vi "mag-field_wait_field.vi"(10 "instr params":T1={"DACs info"={"FPGA VI Reference"=refnum, "Delay"=0, "Last known values"=[], "sent values"=[], "Secured gate"=[], "lock-in config"={"channel (cl)"={"panel LI"=0, "channel LI"=0}, "frequency (Hz)"=0.0, "amplitude (V)"=0.0}, "DAC_Connection"={"DAC"=[], "DAC_Number"=0.0}}, "AWG 8257"={"RF parms"={"Freq(GHz)"={"from"=0.0, "to"=0.0, "String"="", "type"=enum."static"}, "Ampl(dBm)"={"from"=0.0, "to"=0.0, "String"="", "type"=enum."static"}}, "RF on?"=FALSE, "RF info"={"RF freq"=0.0, "RF pow"=0.0, "On?"=FALSE}, "GPIB adr"="", "Activate?"=FALSE, "use System decimal point"=FALSE, "way_of_connection"=0, "VISA_address"=""}, "mag fiel params"={"mag field"={"from"=0.0, "to"=0.0, "type"=enum."static"}, "use perm mode"=FALSE, "field info out"={"B field (consigne)"=0.0, "B field"=0.0, "B-field driver (vi reference)"=refnum, "consigne ctrl (driver)"=refnum, "field has arrived (ctrl, driver)"=refnum, "field  (ctrl, driver)"=refnum, "Coil supply"=refnum, "GPIB adress"=refnum}, "GPIB adr"="", "driver running?"=FALSE, "ON?"=FALSE, "Coil_Information"={"Max Field 10V Input"=0.0, "Waiting time for 0.5mT step"=0.0, "Dac_Output_Channel"=""}}, "K2000 - 01"={"Range (V) 2"="", "Digits 2"="", "NPLC"="", "NPLC fast"="", "GPIB Address"="", "average"=0, "GPIB - PAD"=0, "Use K2000?"=FALSE}, "K2000 - 02"={"Range (V) 2"="", "Digits 2"="", "NPLC"="", "NPLC fast"="", "GPIB Address"="", "average"=0, "GPIB - PAD"=0, "Use K2000?"=FALSE}, "LeCroy6050A"={"LeCroy6050A"={"VISA resource name"="", "Sources"={"Source 1"={"S1_actived"=FALSE, "Source1"=0}, "Source 2"={"S1_actived"=FALSE, "Source1"=0}, "Source 3"={"S1_actived"=FALSE, "Source1"=0}, "Source 4"={"S1_actived"=FALSE, "Source1"=0}}, "Use LeCroy"=FALSE, "time/div"=0.0, "sampling rate"=0.0}, "Activated channels"=[]}, "fast sequence"={"fast channels"={"fast channel 0"={"panel"=0, "chanel"=0, "dummy"=FALSE}, "fast channel 1"={"panel"=0, "chanel"=0, "dummy"=FALSE}, "fast channel 2"={"panel"=0, "chanel"=0, "dummy"=FALSE}, "fast channel 3"={"panel"=0, "chanel"=0, "dummy"=FALSE}, "fast channel 4"={"panel"=0, "chanel"=0, "dummy"=FALSE}, "fast channel 5"={"panel"=0, "chanel"=0, "dummy"=FALSE}, "fast channel 6"={"panel"=0, "chanel"=0, "dummy"=FALSE}, "fast channel 7"={"panel"=0, "chanel"=0, "dummy"=FALSE}, "fast channel 8"={"panel"=0, "chanel"=0, "dummy"=FALSE}, "fast channel 9"={"panel"=0, "chanel"=0, "dummy"=FALSE}, "fast channel 10"={"panel"=0, "chanel"=0, "dummy"=FALSE}, "fast channel 11"={"panel"=0, "chanel"=0, "dummy"=FALSE}, "fast channel 12"={"panel"=0, "chanel"=0, "dummy"=FALSE}, "fast channel 13"={"panel"=0, "chanel"=0, "dummy"=FALSE}, "fast channel 14"={"panel"=0, "chanel"=0, "dummy"=FALSE}, "fast channel 15"={"panel"=0, "chanel"=0, "dummy"=FALSE}}, "Sequence"=[], "used slots"=0, "fast-seq - sweep"={"DACs"=[], "Timings"=[]}, "Num Trigs"=0, "ramp mode"={"ramp"=FALSE, "DACs5"={"DAC"={"name"={"panel"=0, "channel"=0}, "secured 0 ?"=TRUE, "from"=0.0, "to"=0.0, "delta"="", "enabled"=FALSE, "current value"=""}, "DAC 2"={"name"={"panel"=0, "channel"=0}, "secured 0 ?"=TRUE, "from"=0.0, "to"=0.0, "delta"="", "enabled"=FALSE, "current value"=""}, "DAC 3"={"name"={"panel"=0, "channel"=0}, "secured 0 ?"=TRUE, "from"=0.0, "to"=0.0, "delta"="", "enabled"=FALSE, "current value"=""}, "DAC 4"={"name"={"panel"=0, "channel"=0}, "secured 0 ?"=TRUE, "from"=0.0, "to"=0.0, "delta"="", "enabled"=FALSE, "current value"=""}, "DAC 5"={"name"={"panel"=0, "channel"=0}, "secured 0 ?"=TRUE, "from"=0.0, "to"=0.0, "delta"="", "enabled"=FALSE, "current value"=""}, "StartRampAt"=0}}, "fastsequence divider"=0}, "34401A"={"Range (V) 2"="10", "Digits 2"="7", "NPLC"="10", "NPLC fast"="10", "GPIB Address"="", "average"=1, "GPIB - PAD"=0, "Use 34401A?"=FALSE}, "Select Voltmeter"=FALSE, "ArbWG 5014"={"IP adr"="", "RF pulse length"=0, "Channel1 used"=FALSE, "Channel2 used"=FALSE, "Channel3 used"=FALSE, "Channel4 used"=FALSE, "C1_change"={"change1"={"stage"=0.0, "parameters"=0.0, "from"=0.0, "to"=0.0, "type"=enum."static", "waveindex"=0.0}, "change2"={"stage"=0.0, "parameters"=0.0, "from"=0.0, "to"=0.0, "type"=enum."static", "waveindex"=0.0}, "change3"={"stage"=0.0, "parameters"=0.0, "from"=0.0, "to"=0.0, "type"=enum."static", "waveindex"=0.0}, "change4"={"stage"=0.0, "parameters"=0.0, "from"=0.0, "to"=0.0, "type"=enum."static", "waveindex"=0.0}, "change5"={"stage"=0.0, "parameters"=0.0, "from"=0.0, "to"=0.0, "type"=enum."static", "waveindex"=0.0}, "change6"={"stage"=0.0, "parameters"=0.0, "from"=0.0, "to"=0.0, "type"=enum."static", "waveindex"=0.0}, "C1_phase"={"type"=enum."static", "from"=0.0, "to"=0.0}}, "C2_change"={"change1"={"stage"=0.0, "parameters"=0.0, "from"=0.0, "to"=0.0, "type"=enum."static", "waveindex"=0.0}, "change2"={"stage"=0.0, "parameters"=0.0, "from"=0.0, "to"=0.0, "type"=enum."static", "waveindex"=0.0}, "change3"={"stage"=0.0, "parameters"=0.0, "from"=0.0, "to"=0.0, "type"=enum."static", "waveindex"=0.0}, "change4"={"stage"=0.0, "parameters"=0.0, "from"=0.0, "to"=0.0, "type"=enum."static", "waveindex"=0.0}, "change5"={"stage"=0.0, "parameters"=0.0, "from"=0.0, "to"=0.0, "type"=enum."static", "waveindex"=0.0}, "change6"={"stage"=0.0, "parameters"=0.0, "from"=0.0, "to"=0.0, "type"=enum."static", "waveindex"=0.0}, "C2_phase"={"type"=enum."static", "from"=0.0, "to"=0.0}}, "C3_change"={"change1"={"stage"=0.0, "parameters"=0.0, "from"=0.0, "to"=0.0, "type"=enum."static", "waveindex"=0.0}, "change2"={"stage"=0.0, "parameters"=0.0, "from"=0.0, "to"=0.0, "type"=enum."static", "waveindex"=0.0}, "change3"={"stage"=0.0, "parameters"=0.0, "from"=0.0, "to"=0.0, "type"=enum."static", "waveindex"=0.0}, "change4"={"stage"=0.0, "parameters"=0.0, "from"=0.0, "to"=0.0, "type"=enum."static", "waveindex"=0.0}, "change5"={"stage"=0.0, "parameters"=0.0, "from"=0.0, "to"=0.0, "type"=enum."static", "waveindex"=0.0}, "change6"={"stage"=0.0, "parameters"=0.0, "from"=0.0, "to"=0.0, "type"=enum."static", "waveindex"=0.0}, "C3_phase"={"type"=enum."static", "from"=0.0, "to"=0.0}}, "C4_change"={"change1"={"stage"=0.0, "parameters"=0.0, "from"=0.0, "to"=0.0, "type"=enum."static", "waveindex"=0.0}, "change2"={"stage"=0.0, "parameters"=0.0, "from"=0.0, "to"=0.0, "type"=enum."static", "waveindex"=0.0}, "change3"={"stage"=0.0, "parameters"=0.0, "from"=0.0, "to"=0.0, "type"=enum."static", "waveindex"=0.0}, "change4"={"stage"=0.0, "parameters"=0.0, "from"=0.0, "to"=0.0, "type"=enum."static", "waveindex"=0.0}, "change5"={"stage"=0.0, "parameters"=0.0, "from"=0.0, "to"=0.0, "type"=enum."static", "waveindex"=0.0}, "change6"={"stage"=0.0, "parameters"=0.0, "from"=0.0, "to"=0.0, "type"=enum."static", "waveindex"=0.0}, "C4_phase"={"type"=enum."static", "from"=0.0, "to"=0.0}}, "info"=[], "Filename and path"="", "sequence"=FALSE, "ptime"=0.0, "N_seq"=0.0, "polar_seqsize"=0.0, "Activate?"=FALSE, "Samplingrate"={"smplrate from"=0.0, "smplrate to"=0.0, "type"=enum."static"}}, "ADC_conf"={"Range"=0, "Nchannel"=0.0, "Use ADC"=FALSE, "task out"="", "internal clock"="", "Samplingrate"=0.0, "samples per channel"=0, "Realtime?"=FALSE, "RTavg-points"=0.0, "Buffer_size"=1000000, "NPLCmode?"=FALSE, "NPLC"=0.0, "InpConfig"=10106, "SamplingRatePerChannel"=0.0}} {"ADC_conf"."InpConfig" items=["default"=-1, "RSE"=10083, "NRSE"=10078, "Differential"=10106, "Pseudodifferential"=12529]; "ADC_conf"."Range" items=["+/-10V"=10, "+/-5V"=5, "+/-1V"=1, "+/-0,2V"=0]; "34401A"."average" min=1 max=100 step=1; "LeCroy6050A"."LeCroy6050A"."Sources"."Source 4"."Source1" items=["Channel 1", "Channel 2", "Channel 3", "Channel 4", "Memory 1", "Memory 2", "Memory 3", "Memory 4", "Function 1", "Function 2", "Function 3", "Function 4", "Function 5", "Function 6", "Function 7", "Function 8", "Other"]; "LeCroy6050A"."LeCroy6050A"."Sources"."Source 3"."Source1" items=["Channel 1", "Channel 2", "Channel 3", "Channel 4", "Memory 1", "Memory 2", "Memory 3", "Memory 4", "Function 1", "Function 2", "Function 3", "Function 4", "Function 5", "Function 6", "Function 7", "Function 8", "Other"]; "LeCroy6050A"."LeCroy6050A"."Sources"."Source 2"."Source1" items=["Channel 1", "Channel 2", "Channel 3", "Channel 4", "Memory 1", "Memory 2", "Memory 3", "Memory 4", "Function 1", "Function 2", "Function 3", "Function 4", "Function 5", "Function 6", "Function 7", "Function 8", "Other"]; "LeCroy6050A"."LeCroy6050A"."Sources"."Source 1"."Source1" items=["Channel 1", "Channel 2", "Channel 3", "Channel 4", "Memory 1", "Memory 2", "Memory 3", "Memory 4", "Function 1", "Function 2", "Function 3", "Function 4", "Function 5", "Function 6", "Function 7", "Function 8", "Other"]; "fast sequence"."ramp mode"."DACs5"."DAC 5"."name"."channel" max=7 step=1; "fast sequence"."ramp mode"."DACs5"."DAC 5"."name"."panel" max=7 step=1; "fast sequence"."ramp mode"."DACs5"."DAC 4"."name"."channel" max=7 step=1; "fast sequence"."ramp mode"."DACs5"."DAC 4"."name"."panel" max=7 step=1; "fast sequence"."ramp mode"."DACs5"."DAC 3"."name"."channel" max=7 step=1; "fast sequence"."ramp mode"."DACs5"."DAC 3"."name"."panel" max=7 step=1; "fast sequence"."ramp mode"."DACs5"."DAC 2"."name"."channel" max=7 step=1; "fast sequence"."ramp mode"."DACs5"."DAC 2"."name"."panel" max=7 step=1; "fast sequence"."ramp mode"."DACs5"."DAC"."name"."channel" max=7 step=1; "fast sequence"."ramp mode"."DACs5"."DAC"."name"."panel" max=7 step=1; "fast sequence"."Num Trigs" max=1024; "fast sequence"."fast-seq - sweep"."Timings"."slot#" max=4095; "fast sequence"."fast-seq - sweep"."DACs"."sweep infos"."from" min=-1 max=0.5; "fast sequence"."fast-seq - sweep"."DACs"."sweep infos"."to" min=-1 max=0.5; "fast sequence"."fast-seq - sweep"."DACs"."slot#" max=4095; "fast sequence"."Sequence"."slot#" max=4095; "fast sequence"."Sequence"."DAC"."DAC offset" min=-1 max=0.5; "fast sequence"."Sequence"."DAC"."FastChanNum" max=15 step=1; "fast sequence"."fast channels"."fast channel 15"."chanel" max=7 step=1; "fast sequence"."fast channels"."fast channel 15"."panel" max=7 step=1; "fast sequence"."fast channels"."fast channel 14"."chanel" max=7 step=1; "fast sequence"."fast channels"."fast channel 14"."panel" max=7 step=1; "fast sequence"."fast channels"."fast channel 13"."chanel" max=7 step=1; "fast sequence"."fast channels"."fast channel 13"."panel" max=7 step=1; "fast sequence"."fast channels"."fast channel 12"."chanel" max=7 step=1; "fast sequence"."fast channels"."fast channel 12"."panel" max=7 step=1; "fast sequence"."fast channels"."fast channel 11"."chanel" max=7 step=1; "fast sequence"."fast channels"."fast channel 11"."panel" max=7 step=1; "fast sequence"."fast channels"."fast channel 10"."chanel" max=7 step=1; "fast sequence"."fast channels"."fast channel 10"."panel" max=7 step=1; "fast sequence"."fast channels"."fast channel 9"."chanel" max=7 step=1; "fast sequence"."fast channels"."fast channel 9"."panel" max=7 step=1; "fast sequence"."fast channels"."fast channel 8"."chanel" max=7 step=1; "fast sequence"."fast channels"."fast channel 8"."panel" max=7 step=1; "fast sequence"."fast channels"."fast channel 7"."chanel" max=7 step=1; "fast sequence"."fast channels"."fast channel 7"."panel" max=7 step=1; "fast sequence"."fast channels"."fast channel 6"."chanel" max=7 step=1; "fast sequence"."fast channels"."fast channel 6"."panel" max=7 step=1; "fast sequence"."fast channels"."fast channel 5"."chanel" max=7 step=1; "fast sequence"."fast channels"."fast channel 5"."panel" max=7 step=1; "fast sequence"."fast channels"."fast channel 4"."chanel" max=7 step=1; "fast sequence"."fast channels"."fast channel 4"."panel" max=7 step=1; "fast sequence"."fast channels"."fast channel 3"."chanel" max=7 step=1; "fast sequence"."fast channels"."fast channel 3"."panel" max=7 step=1; "fast sequence"."fast channels"."fast channel 2"."chanel" max=7 step=1; "fast sequence"."fast channels"."fast channel 2"."panel" max=7 step=1; "fast sequence"."fast channels"."fast channel 1"."chanel" max=7 step=1; "fast sequence"."fast channels"."fast channel 1"."panel" max=7 step=1; "fast sequence"."fast channels"."fast channel 0"."chanel" max=7 step=1; "fast sequence"."fast channels"."fast channel 0"."panel" max=7 step=1; "K2000 - 02"."average" min=1 max=100 step=1; "K2000 - 01"."average" min=1 max=100 step=1; "DACs info"."lock-in config"."frequency (Hz)" format="%.26g"; "DACs info"."lock-in config"."amplitude (V)" format="%.14g"; "AWG 8257"."way_of_connection" items=["GPIB", "VISA"]; "AWG 8257"."RF parms"."Ampl(dBm)"."to" min=-30 max=18; "AWG 8257"."RF parms"."Ampl(dBm)"."from" min=-30 max=18; "AWG 8257"."RF parms"."Freq(GHz)"."to" min=0.00025 max=20; "AWG 8257"."RF parms"."Freq(GHz)"."from" min=0.00025 max=20}) -> ()   [LabVIEW 2010]
uses:
  type defs - instruments/instruments-params.ctl
  DACs/DAC_info.ctl
  fpga-bitfile-ref.ctl
  DACs/lock-in/lock-in_info.ctl
  DACs/DAC_Connection.ctl
  RF/AWG8257/AWG 8257.ctl
  RF/AWG8257/backend/frequency.ctl
  RF/AWG8257/backend/frequency-limit.ctl
  RF/AWG8257/backend/power.ctl
  RF/AWG8257/backend/power-limits.ctl
  RF/AWG8257/AWG 8257_info.ctl
  mag-field-control.ctl
  type defs - instruments/sweep info.ctl
  type defs - instruments/usage.ctl
  field-info.ctl
  k2000/K2000.ctl
  k2000/k2000 - NPLC.ctl
  le croy 6050A/LeCroy6050A.ctl
  fast sequence/types/fast sequence.ctl
  fast sequence/types/fsatchannels.ctl
  fast sequence/sequence slot/data.ctl
  fast sequence/sequence slot/slot-use.ctl
  fast sequence/sequence slot/triggers.ctl
  fast sequence/sequence slot/DAC.ctl
  fast sequence/sequence slot/DAC_fastseq-offset.ctl
  fast sequence/sequence slot/timing.ctl
  fast sequence/sequence slot/jump.ctl
  fast sequence/sequence - sweep/Data.ctl
  fast sequence/types/sweep info - DAC delta.ctl
  type defs - instruments/sweep info - any.ctl
  DACs/backend/typedefs/DACs5.ctl
  DACs/backend/typedefs/DAC_user.ctl
  DACs/backend/typedefs/panel-channel.ctl
  RF/tektro AWG5014/tektro AWG 5014 - 1.ctl
  ADC/ADC_control.ctl
  fast sequence/sequence slot/slot.xctl
  fast sequence/sequence - sweep/fast-seq - sweep.xctl
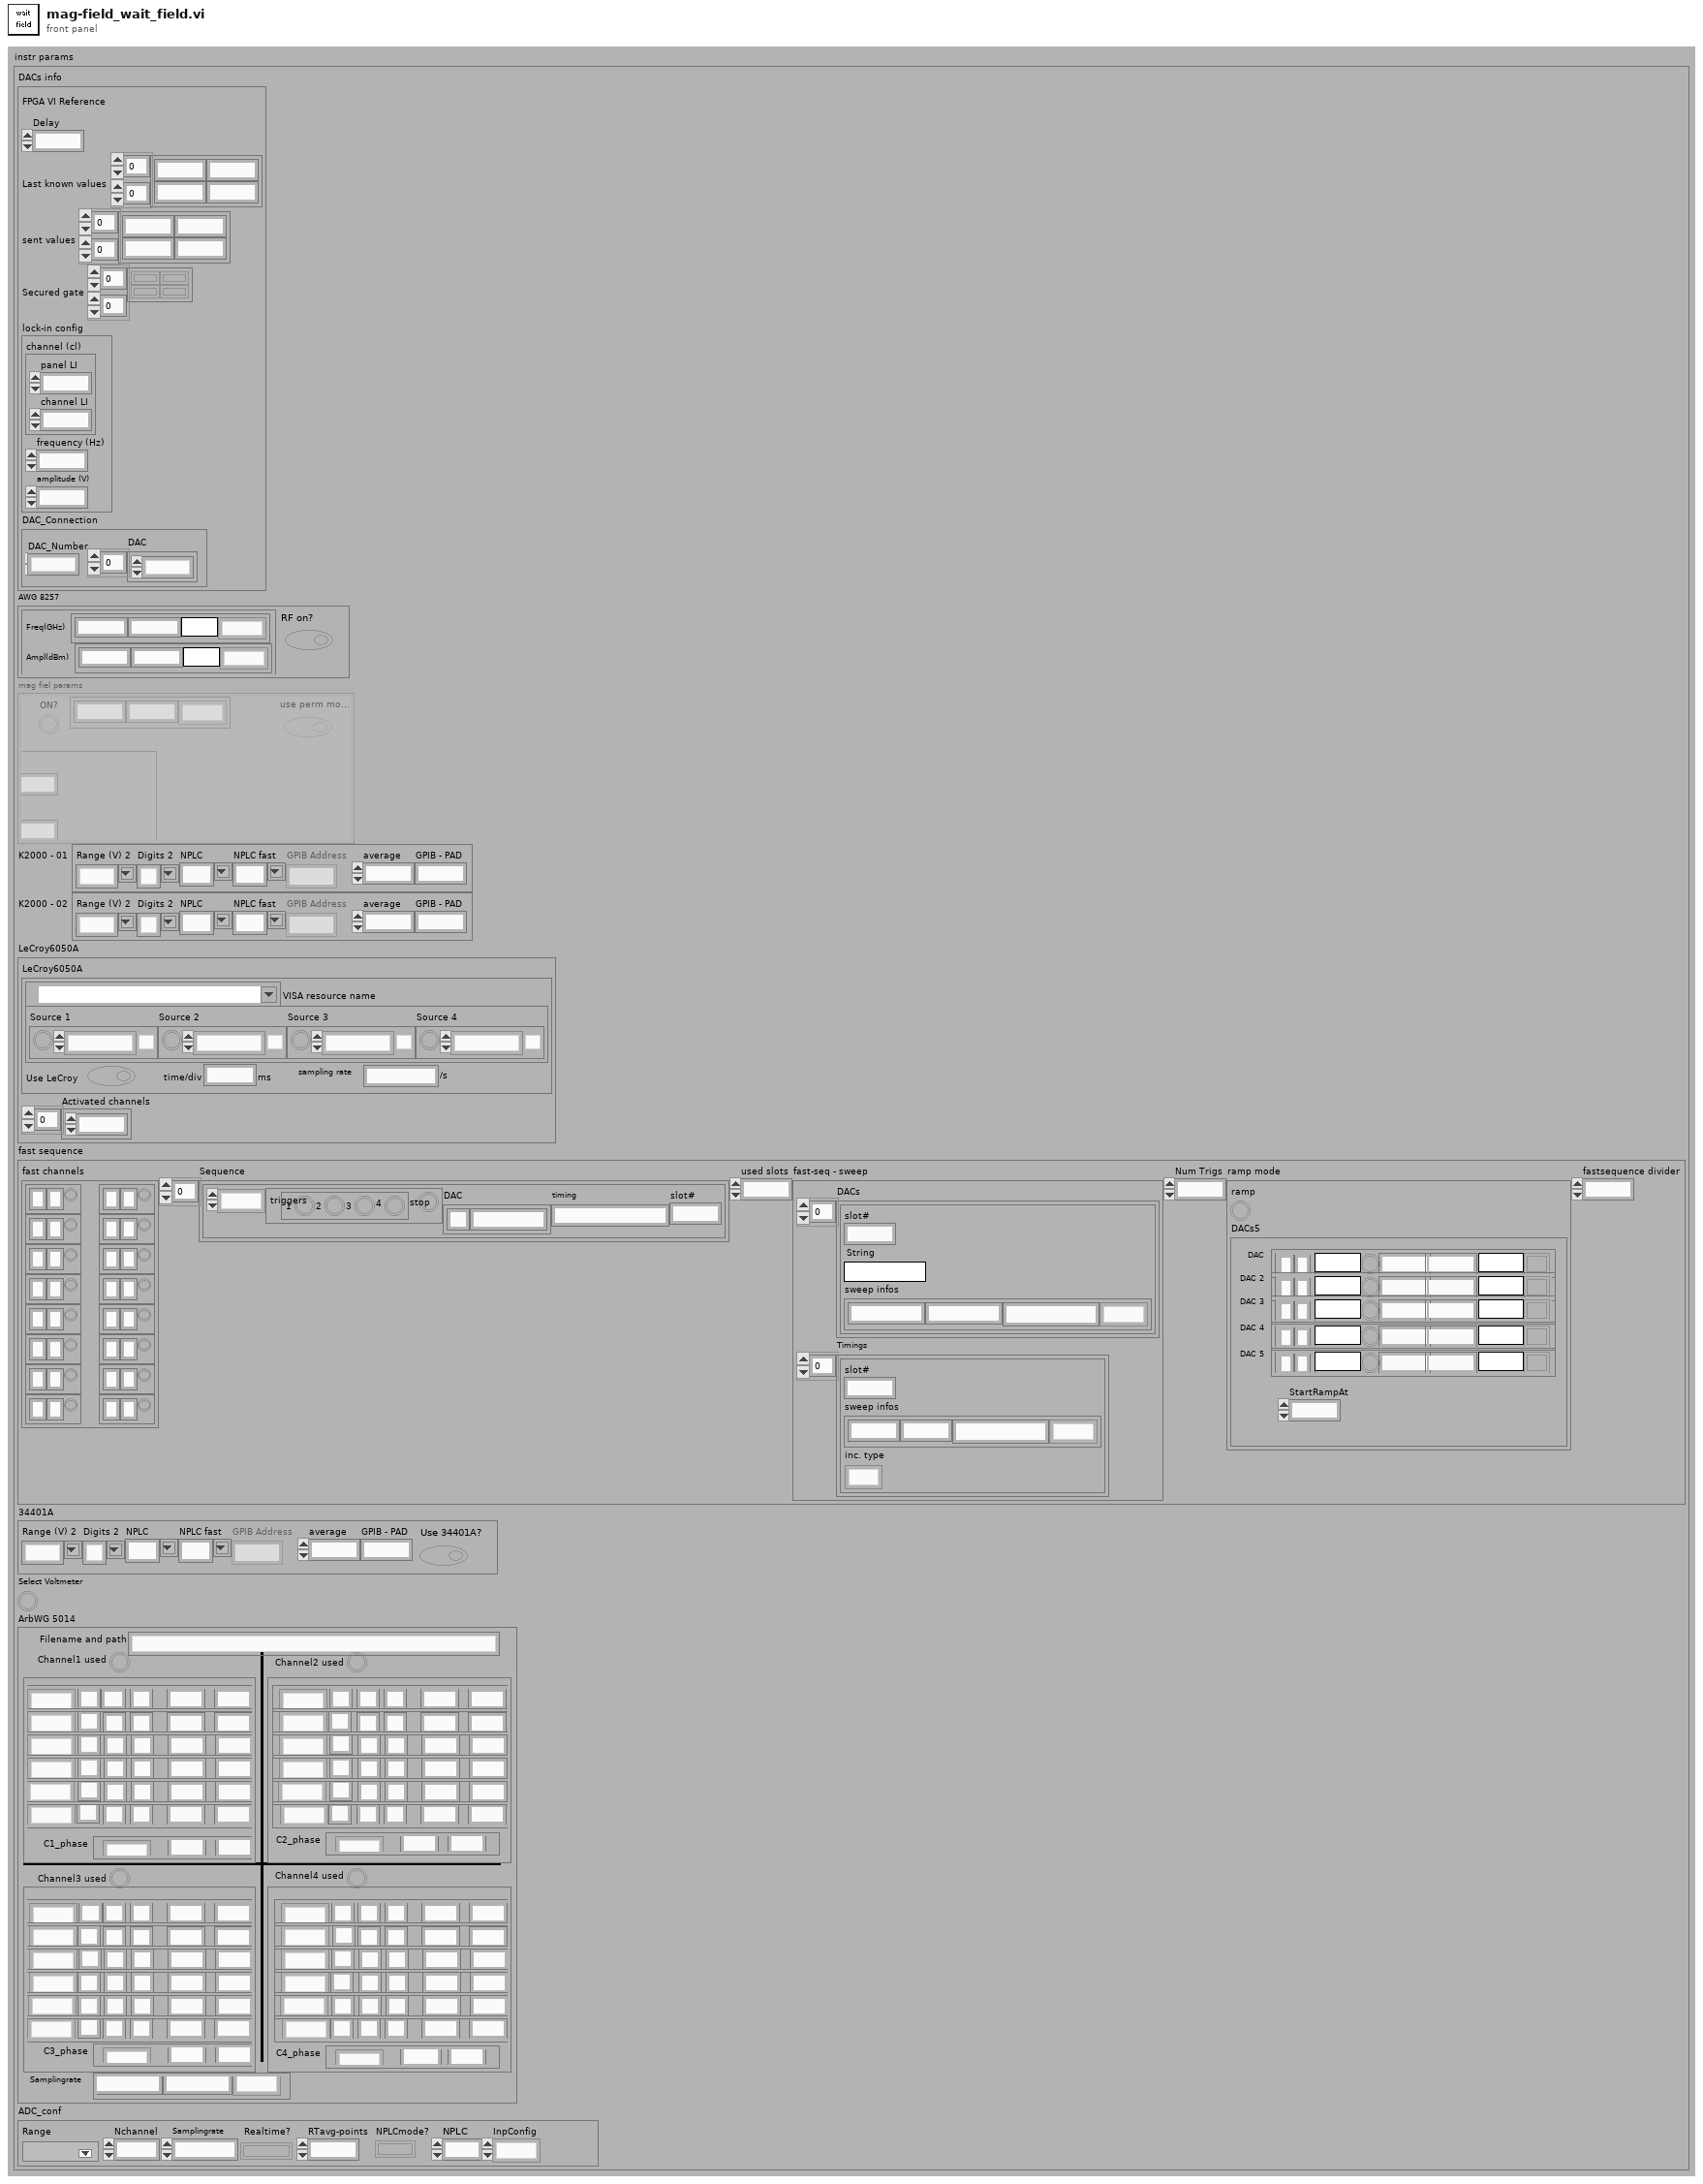
[diagram p1: front panel]
types:
  T1 = typedef "instruments-params.ctl" = cluster{"DACs info":T2, "AWG 8257":T6, "mag fiel params":T12, "K2000 - 01":T16, "K2000 - 02":T16, "LeCroy6050A":cluster{"LeCroy6050A":T18, "Activated channels":u16[]}, "fast sequence":T19, "34401A":cluster{"Range (V) 2":string, "Digits 2":string, "NPLC":string, "NPLC fast":string, "GPIB Address":string, "average":u8, "GPIB - PAD":u8, "Use 34401A?":bool}, "Select Voltmeter":bool, "ArbWG 5014":T34, "ADC_conf":T35}
  T2 = typedef "DAC_info.ctl" = cluster{"FPGA VI Reference":T3, "Delay":u8, "Last known values":dbl[][], "sent values":dbl[][], "Secured gate":bool[][], "lock-in config":T4, "DAC_Connection":T5}
  T3 = typedef "fpga-bitfile-ref.ctl" = refnum<k20>
  T4 = typedef "lock-in_info.ctl" = cluster{"channel (cl)":cluster{"panel LI":u8, "channel LI":u8}, "frequency (Hz)":fxp<+,32,10>, "amplitude (V)":fxp<+,16,3>}
  T5 = typedef "DAC_Connection.ctl" = cluster{"DAC":dbl[], "DAC_Number":dbl}
  T6 = typedef "AWG 8257.ctl" = cluster{"RF parms":cluster{"Freq(GHz)":T7, "Ampl(dBm)":T9}, "RF on?":bool, "RF info":T11, "GPIB adr":string, "Activate?":bool, "use System decimal point":bool, "way_of_connection":u16, "VISA_address":refnum<visa-resource-name>}
  T7 = typedef "frequency.ctl" = cluster{"from":T8, "to":T8, "String":string, "type":enum8{"static", "sweep", "step", "step 2"}}
  T8 = typedef "frequency-limit.ctl" = sgl
  T9 = typedef "power.ctl" = cluster{"from":T10, "to":T10, "String":string, "type":enum8{"static", "sweep", "step", "step 2"}}
  T10 = typedef "power-limits.ctl" = sgl
  T11 = typedef "AWG 8257_info.ctl" = cluster{"RF freq":dbl, "RF pow":dbl, "On?":bool}
  T12 = typedef "mag-field-control.ctl" = cluster{"mag field":T13, "use perm mode":bool, "field info out":T15, "GPIB adr":string, "driver running?":bool, "ON?":bool, "Coil_Information":cluster{"Max Field 10V Input":dbl, "Waiting time for 0.5mT step":dbl, "Dac_Output_Channel":tag}}
  T13 = typedef "sweep info.ctl" = cluster{"from":sgl, "to":sgl, "type":T14}
  T14 = typedef "usage.ctl" = enum8{"static", "sweep", "step", "step 2", "step 3"}
  T15 = typedef "field-info.ctl" = cluster{"B field (consigne)":dbl, "B field":dbl, "B-field driver (vi reference)":refnum<vi>, "consigne ctrl (driver)":refnum<vi>, "field has arrived (ctrl, driver)":refnum<vi>, "field  (ctrl, driver)":refnum<vi>, "Coil supply":refnum<vi>, "GPIB adress":refnum<vi>}
  T16 = typedef "K2000.ctl" = cluster{"Range (V) 2":string, "Digits 2":string, "NPLC":T17, "NPLC fast":T17, "GPIB Address":string, "average":u8, "GPIB - PAD":u8, "Use K2000?":bool}
  T17 = typedef "k2000 - NPLC.ctl" = string
  T18 = typedef "LeCroy6050A.ctl" = cluster{"VISA resource name":refnum<visa-resource-name>, "Sources":cluster{"Source 1":cluster{"S1_actived":bool, "Source1":u16}, "Source 2":cluster{"S1_actived":bool, "Source1":u16}, "Source 3":cluster{"S1_actived":bool, "Source1":u16}, "Source 4":cluster{"S1_actived":bool, "Source1":u16}}, "Use LeCroy":bool, "time/div":sgl[unit], "sampling rate":dbl[unit]}
  T19 = typedef "fast sequence.ctl" = cluster{"fast channels":T20, "Sequence":T21[], "used slots":u8, "fast-seq - sweep":T28, "Num Trigs":u16, "ramp mode":cluster{"ramp":bool, "DACs5":T31}, "fastsequence divider":i32}
  T20 = typedef "fsatchannels.ctl" = cluster{"fast channel 0":cluster{"panel":u8, "chanel":u8, "dummy":bool}, "fast channel 1":cluster{"panel":u8, "chanel":u8, "dummy":bool}, "fast channel 2":cluster{"panel":u8, "chanel":u8, "dummy":bool}, "fast channel 3":cluster{"panel":u8, "chanel":u8, "dummy":bool}, "fast channel 4":cluster{"panel":u8, "chanel":u8, "dummy":bool}, "fast channel 5":cluster{"panel":u8, "chanel":u8, "dummy":bool}, "fast channel 6":cluster{"panel":u8, "chanel":u8, "dummy":bool}, "fast channel 7":cluster{"panel":u8, "chanel":u8, "dummy":bool}, "fast channel 8":cluster{"panel":u8, "chanel":u8, "dummy":bool}, "fast channel 9":cluster{"panel":u8, "chanel":u8, "dummy":bool}, "fast channel 10":cluster{"panel":u8, "chanel":u8, "dummy":bool}, "fast channel 11":cluster{"panel":u8, "chanel":u8, "dummy":bool}, "fast channel 12":cluster{"panel":u8, "chanel":u8, "dummy":bool}, "fast channel 13":cluster{"panel":u8, "chanel":u8, "dummy":bool}, "fast channel 14":cluster{"panel":u8, "chanel":u8, "dummy":bool}, "fast channel 15":cluster{"panel":u8, "chanel":u8, "dummy":bool}}
  T21 = typedef "slot.xctl/data.ctl" = cluster{"use":T22, "Triggers":T23, "DAC":T24, "timing":T26, "slot#":T27}
  T22 = typedef "slot-use.ctl" = enum8{"DAC", "timing", "triggers", "jump"}
  T23 = typedef "triggers.ctl" = cluster{"triggers":cluster{"1":bool, "2":bool, "3":bool, "4":bool}, "stop":bool}
  T24 = typedef "DAC.ctl" = cluster{"FastChanNum":u8, "DAC offset":T25}
  T25 = typedef "DAC_fastseq-offset.ctl" = sgl
  T26 = typedef "timing.ctl" = sgl
  T27 = typedef "jump.ctl" = u16
  T28 = typedef "fast-seq - sweep.xctl/Data.ctl" = cluster{"DACs":cluster{"slot#":T27, "String":string, "sweep infos":T29}[], "Timings":cluster{"slot#":T27, "sweep infos":T30, "inc. type":enum16{"flat", "inc.", "dec"}}[]}
  T29 = typedef "sweep info - DAC delta.ctl" = cluster{"from":T25, "to":T25, "String":string, "type":T14}
  T30 = typedef "sweep info - any.ctl" = cluster{"from":sgl, "to":sgl, "String":string, "type":T14}
  T31 = typedef "DACs5.ctl" = cluster{"DAC":T32, "DAC 2":T32, "DAC 3":T32, "DAC 4":T32, "DAC 5":T32, "StartRampAt":u8}
  T32 = typedef "DAC_user.ctl" = cluster{"name":T33, "secured 0 ?":bool, "from":sgl, "to":sgl, "delta":string, "enabled":bool, "current value":string}
  T33 = typedef "panel-channel.ctl" = cluster{"panel":u8, "channel":u8}
  T34 = typedef "tektro AWG 5014 - 1.ctl" = cluster{"IP adr":string, "RF pulse length":u16, "Channel1 used":bool, "Channel2 used":bool, "Channel3 used":bool, "Channel4 used":bool, "C1_change":cluster{"change1":cluster{"stage":sgl, "parameters":sgl, "from":sgl, "to":sgl, "type":T14, "waveindex":dbl}, "change2":cluster{"stage":sgl, "parameters":sgl, "from":sgl, "to":sgl, "type":T14, "waveindex":dbl}, "change3":cluster{"stage":sgl, "parameters":sgl, "from":sgl, "to":sgl, "type":T14, "waveindex":dbl}, "change4":cluster{"stage":sgl, "parameters":sgl, "from":sgl, "to":sgl, "type":T14, "waveindex":dbl}, "change5":cluster{"stage":sgl, "parameters":sgl, "from":sgl, "to":sgl, "type":T14, "waveindex":dbl}, "change6":cluster{"stage":sgl, "parameters":sgl, "from":sgl, "to":sgl, "type":T14, "waveindex":dbl}, "C1_phase":cluster{"type":T14, "from":sgl, "to":sgl}}, "C2_change":cluster{"change1":cluster{"stage":sgl, "parameters":sgl, "from":sgl, "to":sgl, "type":T14, "waveindex":dbl}, "change2":cluster{"stage":sgl, "parameters":sgl, "from":sgl, "to":sgl, "type":T14, "waveindex":dbl}, "change3":cluster{"stage":sgl, "parameters":sgl, "from":sgl, "to":sgl, "type":T14, "waveindex":dbl}, "change4":cluster{"stage":sgl, "parameters":sgl, "from":sgl, "to":sgl, "type":T14, "waveindex":dbl}, "change5":cluster{"stage":sgl, "parameters":sgl, "from":sgl, "to":sgl, "type":T14, "waveindex":dbl}, "change6":cluster{"stage":sgl, "parameters":sgl, "from":sgl, "to":sgl, "type":T14, "waveindex":dbl}, "C2_phase":cluster{"type":T14, "from":sgl, "to":sgl}}, "C3_change":cluster{"change1":cluster{"stage":sgl, "parameters":sgl, "from":sgl, "to":sgl, "type":T14, "waveindex":dbl}, "change2":cluster{"stage":sgl, "parameters":sgl, "from":sgl, "to":sgl, "type":T14, "waveindex":dbl}, "change3":cluster{"stage":sgl, "parameters":sgl, "from":sgl, "to":sgl, "type":T14, "waveindex":dbl}, "change4":cluster{"stage":sgl, "parameters":sgl, "from":sgl, "to":sgl, "type":T14, "waveindex":dbl}, "change5":cluster{"stage":sgl, "parameters":sgl, "from":sgl, "to":sgl, "type":T14, "waveindex":dbl}, "change6":cluster{"stage":sgl, "parameters":sgl, "from":sgl, "to":sgl, "type":T14, "waveindex":dbl}, "C3_phase":cluster{"type":T14, "from":sgl, "to":sgl}}, "C4_change":cluster{"change1":cluster{"stage":sgl, "parameters":sgl, "from":sgl, "to":sgl, "type":T14, "waveindex":dbl}, "change2":cluster{"stage":sgl, "parameters":sgl, "from":sgl, "to":sgl, "type":T14, "waveindex":dbl}, "change3":cluster{"stage":sgl, "parameters":sgl, "from":sgl, "to":sgl, "type":T14, "waveindex":dbl}, "change4":cluster{"stage":sgl, "parameters":sgl, "from":sgl, "to":sgl, "type":T14, "waveindex":dbl}, "change5":cluster{"stage":sgl, "parameters":sgl, "from":sgl, "to":sgl, "type":T14, "waveindex":dbl}, "change6":cluster{"stage":sgl, "parameters":sgl, "from":sgl, "to":sgl, "type":T14, "waveindex":dbl}, "C4_phase":cluster{"type":T14, "from":sgl, "to":sgl}}, "info":sgl[][][][], "Filename and path":string, "sequence":bool, "ptime":dbl, "N_seq":dbl, "polar_seqsize":dbl, "Activate?":bool, "Samplingrate":cluster{"smplrate from":dbl, "smplrate to":dbl, "type":T14}}
  T35 = typedef "ADC_control.ctl" = cluster{"Range":i16, "Nchannel":dbl, "Use ADC":bool, "task out":refnum<k21>, "internal clock":refnum<k21>, "Samplingrate":dbl, "samples per channel":u32, "Realtime?":bool, "RTavg-points":dbl, "Buffer_size":i32, "NPLCmode?":bool, "NPLC":dbl, "InpConfig":i32, "SamplingRatePerChannel":dbl}
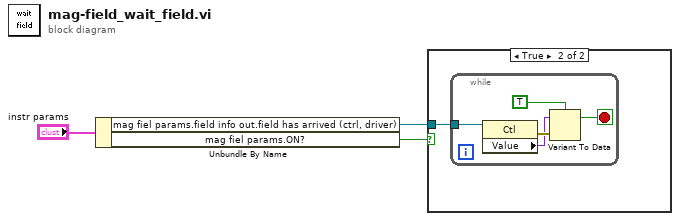
[diagram p0: block diagram]
diagram:
  n1 = Unbundle By Name("instr params") -> ("mag fiel params.field info out.field has arrived (ctrl, driver)"=w2:refnum<vi>, "mag fiel params.ON?"=w1:bool)
  n2 = case shown="True" w1 {
    tunnel: w2 -> [_ w4]
    frame False {
    }
    frame True {
      n3 = while {
        tunnel: w4 -> [w9]
        stop <- w5 stop-if-true
        n4 = property class="Ctl"(reference=w9) -> (error out=w8:errorcluster, "Value"=w7:variant)  [unwired: 1 in, 1 out]
        n5 = Variant To Data(error in=w8, Variant=w7, type=TRUE) -> (data=w5:bool)  [unwired: 1 out]
      }
    }
  }
